vi "Elution_stop.vi"() -> ()   [LabVIEW 2021]
panel:
  out "Elution_stop":bool
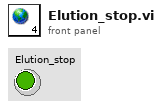
[diagram p1: front panel]
diagram:
